vi "Vision (SubVI).vi"(11 "stop":bool) -> (0 "error out":errorcluster, 1 "GREEN?":bool, 2 "RED?":bool, 3 "Iteration Duration":i64)   [LabVIEW 2017]
uses:
  <vilib>/Platform/TimedLoop/XDataNode/timing_clust.ctl
  <vilib>/Platform/TimedLoop/XDataNode/nitl_modes.ctl
  <vilib>/Platform/TimedLoop/XDataNode/wakeup.ctl
  <vilib>/Platform/TimedLoop/XDataNode/XDataNode.xnode
  <vilib>/Platform/TimedLoop/XDataNode/XDNodeRunTimeDep.lvlib
panel:
  out "x .or. y?":bool
  out "element 2":dbl
  out "element":dbl
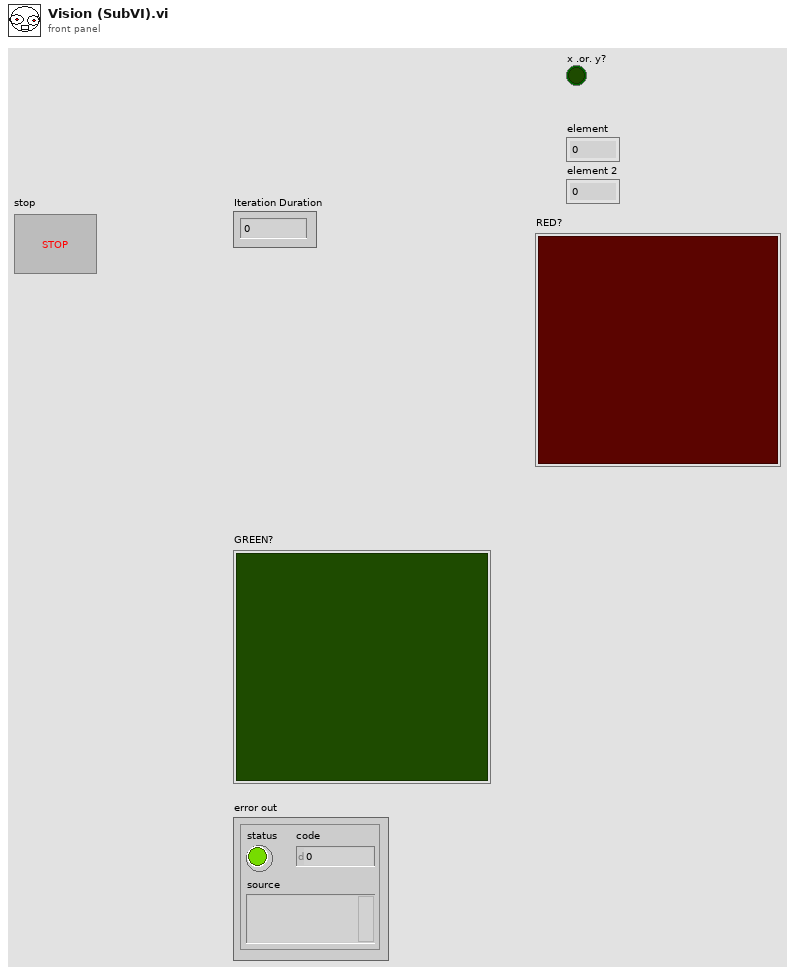
[diagram p1: front panel]
types:
  T1 = typedef "XDNodeRunTimeDep.lvlib/timing_clust.ctl" = cluster{"Expected End [f-1]":u64, "Actual End [f-1]":u64, "Finished Late? [f-1]":bool, "Expected End [i-1]":u64, "Actual End [i-1]":u64, "Finished Late? [i-1]":bool, "Expected Start [i]":u64, "Actual Start [i]":u64, "Expected Start [f]":u64, "Actual Start [f]":u64, "Source Name":string, "Structure Name":string, "Period":i64, "Deadline":i64, "Offset":i64, "Start":i64, "Priority":i32, "Timeout":i32, "Mode":T2, "Wakeup Reason":T3, "Error":errorcluster, "Source Type":string, "Secondary Source Type":string, "Global End Time":u64, "Global Start Time":u64, "Frame Duration":u64, "Iteration Duration":u64, "Assigned CPU":i32, "I/O Scan Engine Mode":u32}
  T2 = typedef "XDNodeRunTimeDep.lvlib/nitl_modes.ctl" = enum32{"No Change", "Process missed periods, maintain original phase", "Discard missed periods, maintain original phase", "Process missed periods, ignore original phase", "Discard missed periods, ignore original phase"}
  T3 = typedef "XDNodeRunTimeDep.lvlib/wakeup.ctl" = enum32{"Normal", "Aborted", "Asynchronous wakeup", "Timing source error", "Timed loop error", "Timeout"}
  T4 = typedef "IMAQ Image.ctl" = refnum<image>
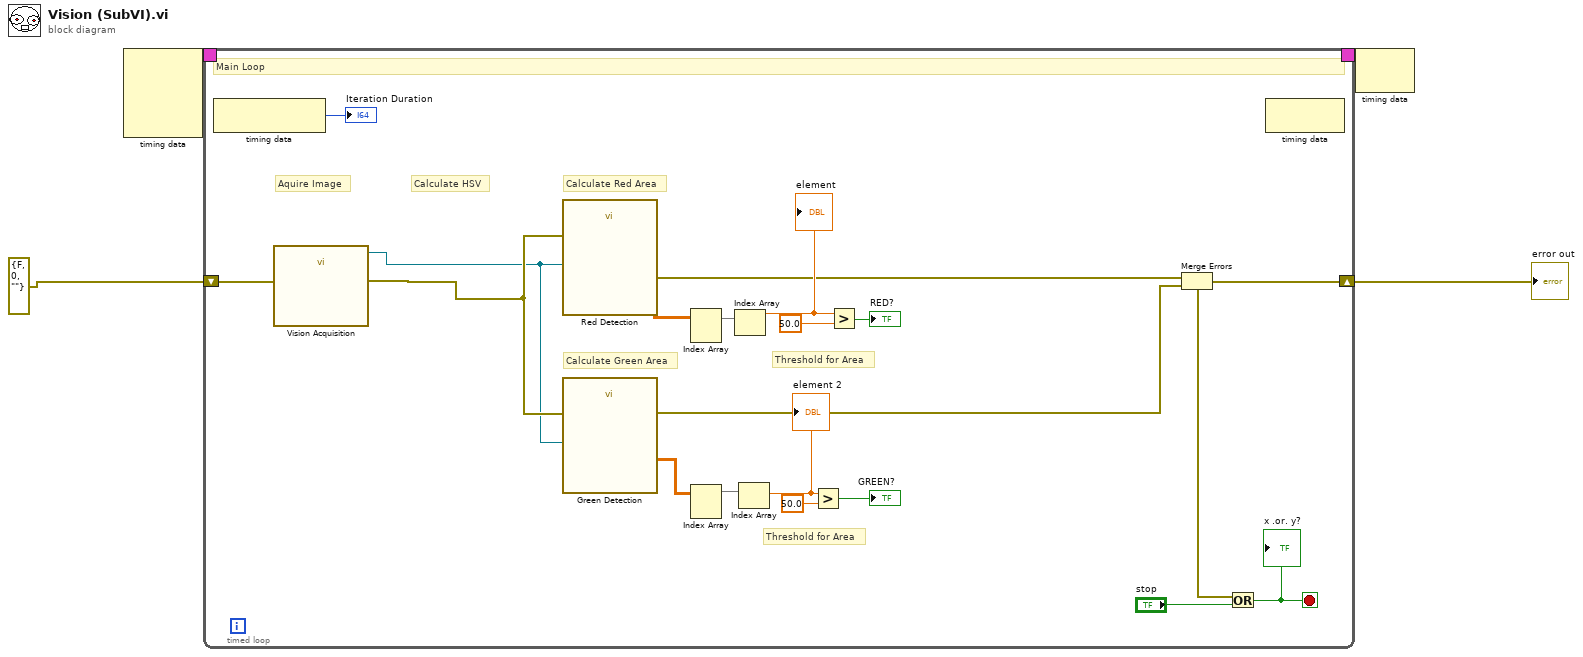
[diagram p0: block diagram]
diagram:
  n1 = node-c288() -> (w2:T1)  [unwired: 4 in]
  n2 = timed-loop {
    shift-right: [w8] -> w3
    shift-left: errorcluster {"status"=FALSE, "code"=0, "source"=""} ("error in (no error)") -> [w23]
    timing: w2 -> [_]
    timing-out: [_] -> w1
    stop <- w7 stop-if-true
    # "Calculate Green Area"
    # "Calculate Red Area"
    # "Calculate HSV"
    # "Aquire Image"
    # "Threshold for Area"
    # "Threshold for Area"
    # "Main Loop"
    n3 = node-c288() -> (→"Iteration Duration":i64)  [unwired: 1 in]
    n4 = call "Vision Acquisition"("error in"=w23) -> ("Image Out"=w5:T4, "error out"=w6:errorcluster)  [unwired: 24 in, 1 out]
    n5 = call "Red Detection"("Image In"=w5, "error in"=w6) -> ("Particle Measurements (Pixels) (Particle Analysis 1)"=w18:dbl[][], "error out"=w10:errorcluster)  [unwired: 23 in, 1 out]
    n6 = call "Green Detection"("Image In"=w5, "error in"=w6) -> ("Particle Measurements (Pixels) (Particle Analysis 1)"=w14:dbl[][], "error out"=w9:errorcluster)  [unwired: 23 in, 1 out]
    n7 = Index Array(array=w18) -> (element=w12:dbl[])  [unwired: 2 in]
    n8 = Index Array(array=w14) -> (element=w17:dbl[])  [unwired: 2 in]
    n9 = Index Array(array=w12) -> (element=w22:dbl)  [unwired: 1 in]
    "element" <- w22
    n10 = Index Array(array=w17) -> (element=w16:dbl)  [unwired: 1 in]
    "element 2" <- w16
    n11 = Greater?(x=w16, y=50.0) -> (0:→"GREEN?":bool)
    n12 = Greater?(x=w22, y=50.0) -> (0:→"RED?":bool)
    n13 = Merge Errors(w10, w9) -> (w8:errorcluster)
    n14 = Or(x=w8, y="stop") -> (x .or. y?=w7:bool)
    "x .or. y?" <- w7
    n15 = node-c288() -> ()  [unwired: 1 in, 1 out]
  }
  "error out" <- w3
  n16 = node-c288(w1) -> ()  [unwired: 1 out]
